vi "Exercise 1.7.vi"() -> ()   [LabVIEW 2010]
panel:
  out "Result 1":dbl
  out "Result 2":dbl
  in  "Number 4":dbl
  in  "Number 6":dbl
  in  "Number 5":dbl
  in  "Number 3":dbl
  in  "Number 2":dbl
  in  "Number 1":dbl
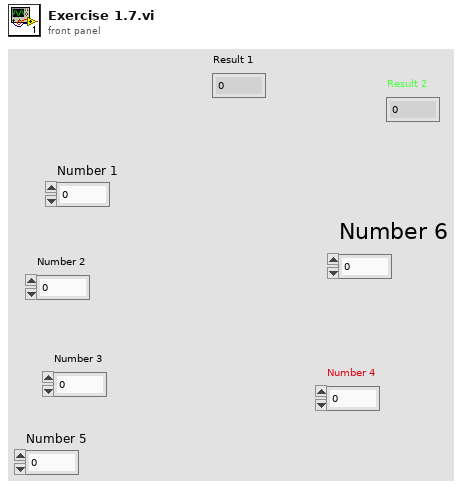
[diagram p1: front panel]
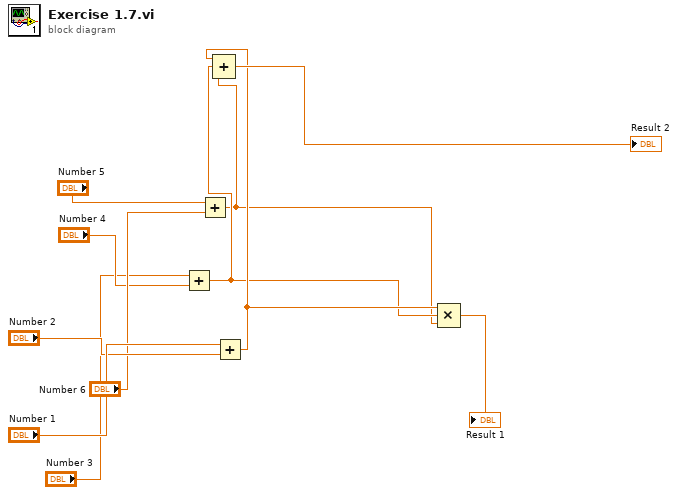
[diagram p0: block diagram]
diagram:
  n1 = Add(x="Number 3", y="Number 4") -> (x+y=w3:dbl)
  n2 = Add(x="Number 5", y="Number 6") -> (x+y=w2:dbl)
  n3 = Add(x="Number 1", y="Number 2") -> (x+y=w4:dbl)
  n4 = Compound Arithmetic op=ADD(w4, w3, w2) -> (→"Result 2":dbl)
  n5 = Compound Arithmetic op=MULTIPLY(w4, w3, w2) -> (→"Result 1":dbl)
